vi "Create Bitfile.vi"(8 "error in (no error)":errorcluster, 9 "Bitfile Path in":path, 10 "RIO Device Address in":string, 11 "Item Ref in":T1 format="%.0x") -> (0 "error out":errorcluster, 2 "RIO Addresses":string[](array[string]), 3 "Item Ref out":T1 format="%.0x")   [LabVIEW 2015, in "Engine Simulation Toolkit System Explorer.lvlib"]
uses:
  Engine Simulation Toolkit System Explorer.lvlib
  <vilib>/NI Veristand/Custom Device API/Custom Device Item Ref.ctl
  Shared/Properties.vi
  <vilib>/NI Veristand/Custom Device API/Get Item Property (String Array).vi
  <vilib>/NI Veristand/Custom Device API/Set Item Property (String Array).vi
  Shared/Engine Simulation Toolkit Shared.lvlib
  <vilib>/NI VeriStand/Custom Device API/Custom Device API.lvlib
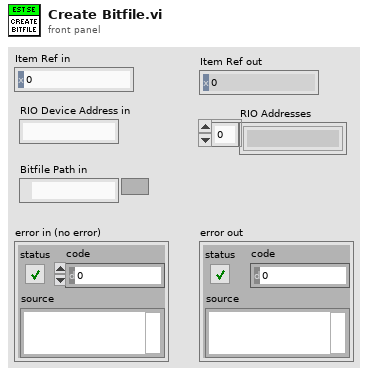
[diagram p1: front panel]
types:
  T1 = typedef "Custom Device API.lvlib/Custom Device Item Ref.ctl" = u64
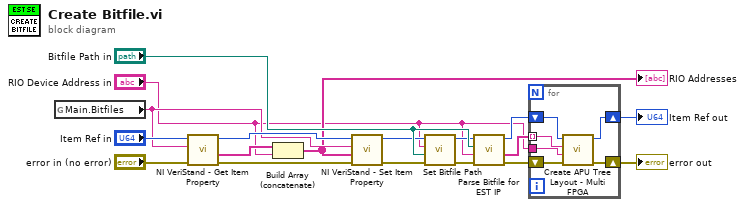
[diagram p0: block diagram]
diagram:
  n1 = global read "Properties.vi" "Main.Bitfiles"() -> (w4:string)
  n2 = call-poly <vilib>:"NI VeriStand - Get Item Property.vi"("error in (no error)"="error in (no error)", "Property Name"=w4, "Item Ref in"="Item Ref in") -> ("error out"=w6:errorcluster, "Value"=w2:string[], "Item Ref out"=w7:T1)  [unwired: 5 in, 1 out]
  n3 = Build Array (concatenate)(w2, "RIO Device Address in") -> (w3:string[])
  "RIO Addresses" <- w3
  n4 = call-poly <vilib>:"NI VeriStand - Set Item Property.vi"("error in (no error)"=w6, "Value"=w3, "Property Name"=w4, "Item Ref in"=w7) -> ("error out"=w10:errorcluster, "Item Ref out"=w9:T1)  [unwired: 5 in, 1 out]
  n5 = call "Set Bitfile Path.vi"("error in (no error)"=w10, "Bitfile Path in"="Bitfile Path in", "RIO Device Address in"="RIO Device Address in", "Item Ref in"=w9) -> ("error out"=w12:errorcluster, "Item Ref out"=w13:T1)  [unwired: 6 in]
  n6 = call "Parse Bitfile for EST IP.vi"("error in (no error)"=w12, "RIO device address"="RIO Device Address in", "bitfile path"="Bitfile Path in", "Item Ref in"=w13) -> ("error out"=w16:errorcluster, "APUs"=w17:string[], "Item Ref out"=w18:T1)  [unwired: 4 in, 1 out]
  n7 = for {
    shift-right: [w23] -> w11
    shift-left: w16 -> [w24]
    tunnel: w17 -> [w21] mode=indexing
    tunnel: "RIO Device Address in" -> [w20]
    shift-right: [w19] -> w14
    shift-left: w18 -> [w22]
    n8 = call "Create APU Tree Layout - Multi FPGA.vi"("error in (no error)"=w24, "rio name"=w20, "engine name"=w21, "Section Ptr"=w22) -> ("error out"=w23:errorcluster, "Section Ptr dup"=w19:T1)  [unwired: 5 in, 1 out]
  }
  "error out" <- w11
  "Item Ref out" <- w14
